vi "getReferenceDomainOffset.vi"(8 "error in (no error)":errorcluster, 11 "IReferenceDomainInfo in":refnum<class "IReferenceDomainInfo.lvclass">) -> (0 "error out":errorcluster, 2 "DomainOffset out":i32, 3 "IReferenceDomainInfo out":refnum<class "IReferenceDomainInfo.lvclass">)   [LabVIEW 2022 SP3, in "openDAQ.lvlib" / "IBaseObject.lvlib" / "IReferenceDomainInfo.lvlib" / "IReferenceDomainInfo.lvclass"]
uses:
  <instrlib>/openDAQ/Public/Classes/IReferenceDomainInfo/IReferenceDomainInfo.lvclass
  C:/Program Files (x86)/National Instruments/LabVIEW 2022/instr.lib/openDAQ/Public/Classes/IBaseObject/IBaseObject.lvclass
  <instrlib>/openDAQ/Public/Classes/daqCoreTypes/IInteger/IInteger.lvclass
  <instrlib>/openDAQ/Public/Classes/IBaseObject/IBaseObject.lvclass/IBaseObject.ctl
  <instrlib>/openDAQ/Public/Classes/IBaseObject/Accessor/Read reference.vi
  <instrlib>/openDAQ/Public/Classes/IBaseObject/Accessor/Write reference.vi
  <instrlib>/openDAQ/Public/Classes/IReferenceDomainInfo/IReferenceDomainInfo.lvclass/IReferenceDomainInfo.ctl
  <instrlib>/openDAQ/Binaries/Windows/x86/copendaq32.dll
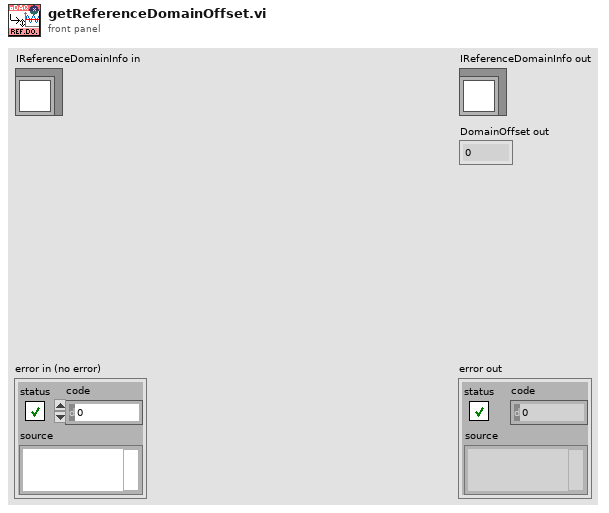
[diagram p1: front panel]
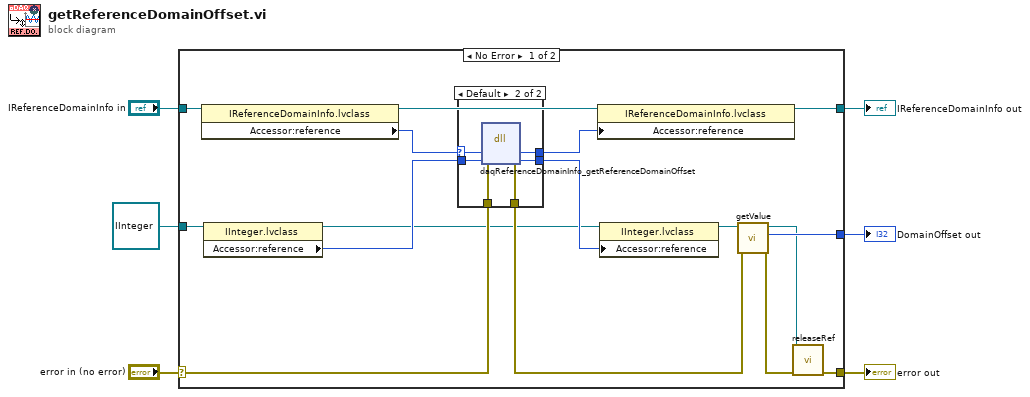
[diagram p0: block diagram]
diagram:
  n1 = case shown="No Error" "error in (no error)" {
    selector: "error in (no error)" -> [w20 w31]
    tunnel: [w10 w31] -> w5
    tunnel: [w18 w30] -> w3
    tunnel: "IReferenceDomainInfo in" -> [w21 w30]
    tunnel: refnum<class "IInteger.lvclass"> refnum ("openDAQ.lvlib:daqCoreTypes.lvlib:IInteger.lvclass") -> [w16 _]
    tunnel: [w22 _] -> w1
    frame No Error {
      n2 = property class="IReferenceDomainInfo.lvclass"(reference=w21) -> (reference out=w19:refnum<class "IReferenceDomainInfo.lvclass">, "Accessor:reference"=w7:i64)  [unwired: 1 in, 1 out]
      n3 = property class="IInteger.lvclass"(reference=w16) -> (reference out=w8:refnum<class "IInteger.lvclass">, "Accessor:reference"=w15:i64)  [unwired: 1 in, 1 out]
      n4 = case shown="Default" w7 {
        selector: w7 -> [_ w24]
        tunnel: w20 -> [w23 w29]
        tunnel: [_ w28] -> w17
        tunnel: w15 -> [_ w27]
        tunnel: [_ w26] -> w14
        tunnel: [w23 w25] -> w12
        frame 0 {
        }
        frame Default {
          n5 = dll-call lib="C:/Program Files (x86)/National Instruments/LabVIEW 2022/instr.lib/openDAQ/Binaries/Windows/x86/copendaq*.*" fn="daqReferenceDomainInfo_getReferenceDomainOffset"(error in=w29, "referenceDomainInfo"=w24, "domainOffset"=w27) -> (error out=w25:errorcluster, "referenceDomainInfo"=w28:i64, "domainOffset"=w26:i64)  [unwired: 3 in, 1 out]
        }
      }
      n6 = property class="IReferenceDomainInfo.lvclass"(reference=w19, "Accessor:reference"=w17) -> (reference out=w18:refnum<class "IReferenceDomainInfo.lvclass">)  [unwired: 1 in, 1 out]
      n7 = property class="IInteger.lvclass"(reference=w8, "Accessor:reference"=w14) -> (reference out=w13:refnum<class "IInteger.lvclass">)  [unwired: 1 in, 1 out]
      n8 = call <instrlib>:"getValue.vi"("error in (no error)"=w12, "IInteger in"=w13) -> ("error out"=w11:errorcluster, "Value out"=w22:i32, "IInteger out"=w9:refnum<class "IInteger.lvclass">)  [unwired: 7 in]
      n9 = call-dynamic "releaseRef.vi"("error in (no error)"=w11, "IBaseObject in"=w9) -> ("error out"=w10:errorcluster)  [unwired: 9 in]
    }
    frame Error {
    }
  }
  "error out" <- w5
  "IReferenceDomainInfo out" <- w3
  "DomainOffset out" <- w1
